vi "Dashboard Main.vi"() -> ()   [LabVIEW 2013]
uses:
  <vilib>/event_ctls.llb/eventvkey.ctl
  <vilib>/Rock Robotics/WPI/Dashboard/WPI_DashboardLogging Global.vi
  <vilib>/Utility/config.llb/Write Key (String).vi
  <vilib>/Utility/config.llb/Write Key (I32).vi
  <vilib>/Utility/config.llb/Read Key (String).vi
  <vilib>/Utility/config.llb/NI_LVConfig.lvlib
panel:
  in  "Save to File":bool
  in  "Read from File":bool=TRUE
  out "Image Message":string="Timeout in Camera Communications"
  in  "Rec Mode":enum32{"Stop", "Record", "Playback"}(radio)
  in  "Dashboard Tab":T1(tab)=enum."Drivetrain"
  in  "Camera Settings":T2={"Frame Rate"=30, "Compression"=30, "Size"=1} {"Frame Rate" scale=1.0..30.0; "Size" items=["640x480", "320x240", "160x120"]}
  out "MotorSliders R":cluster{"MotorSlide1":dbl, "MotorSlide2":dbl} {"MotorSlide2" scale=-1.0..1.0 scale format="%#_2e"; "MotorSlide1" scale=-1.0..1.0 scale format="%#_2e"}
  out "MotorChart R":cluster{"Numeric":dbl, "Numeric":dbl}(graph)
  out "MotorSliders L":T3 {"MotorSlide4 2" scale=0.0..14.0 scale format="%#_2e"; "MotorSlide2" scale=-1.0..1.0 scale format="%#_2e"; "MotorSlide1" scale=-1.0..1.0 scale format="%#_2e"}
  out "MotorChart L":T4(graph)
  out "JS1 Z":dbl(slide) scale=-1.0..1.0 scale format="%#_2e"
  out "Joystick 1":cluster{"X":dbl, "Y":dbl}[](graph)
  out "JS Buttons 1":T5
  out "JS2 Z":dbl(slide) scale=-1.0..1.0 scale format="%#_2e"
  out "Joystick 2":cluster{"X":dbl, "Y":dbl}[](graph)
  out "JS Buttons 2":T5
  out "Mode":T6(ring)=enum.""
  out "Camera IP":string="0.0.0.11"
  in  "DB Camera Config":bool
  out "fps":dbl format="%#.1g"
  out "Mbps":dbl format="%#.1g"
  out "Mbps 2":bool
  out "LED 1":bool
  in  "String":string
  in  "Dial":i8(knob) scale=0.0..10.0
  in  "Slider 1":dbl(slide) scale=0.0..100.0
  in  "Checkbox 2":bool
  in  "Checkbox 1":bool
  in  "Test Slider":dbl(slide) scale=0.0..100.0 scale format="%#_3g"
  in  "On/Off":bool caption="Solenoid"
  in  "Test Name":u16(ring) items=["Select the test to run...", "Example Test", "-------------------------------", "List of tests is built in robot code.", "Replace with your own automated tests."]
  in  "Test Tree":string(tree)
  in  "Motor":cluster{"Value":dbl, "Enable":bool} {"Value" scale=-1.0..1.0 scale format="%#_3g"}
  out "Progress":T7 {"Test Progress" scale=0.0..100.0}
  in  "Rev/Fwd":cluster{"Forward":bool, "Reverse":bool}
  in  "Test Ring":u16(ring) items=["Auto", "Fixed indoor", "Fixed outdoor 1", "Fixed outdoor 2", "Fixed fluorescent 1", "Fixed fluorescent 2", "Hold current"]
  in  "Listbox":i32(listbox)
  out "Tree":string(tree)
  in  "MaxSuspend":dbl=200.0
  in  "MinMotorPower":dbl
  in  "MinJoystickChange":dbl=0.05
  in  "ShiftDelay":dbl=200.0
  in  "DeadZone":dbl=0.1
  out "Camera Image":T8(plugin-control)
  in  "Enable":bool
  # "Left"
  # "Front"
  # "Right"
  # "Battery"
  # "Customize by placing controls and indicators here and name to\nmatch Dashboard Variables on robot."
  # "This tab is a great place for autonomous settings and validation.\nCustomize by placing controls and indicators here and name to\nmatch Dashboard Variables on robot."
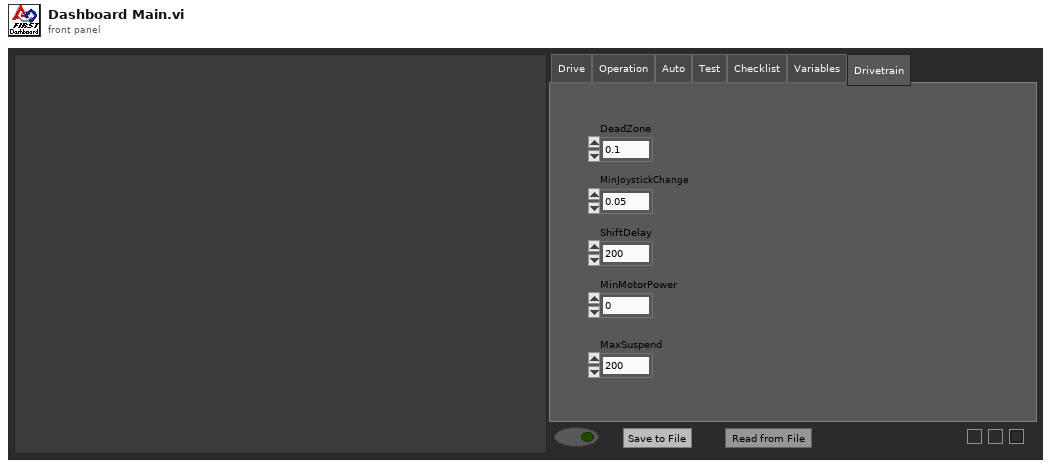
[diagram p1: front panel]
types:
  T1 = enum32{"Drive", "Operation", "Auto", "Test", "Checklist", "Variables", "Drivetrain"}
  T2 = cluster{"Frame Rate":i32, "Compression":i32, "Size":u16}
  T3 = cluster{"MotorSlide1":dbl, "MotorSlide2":dbl, "MotorSlide4 2":dbl}
  T4 = cluster{"Numeric":dbl, "Numeric":dbl, "Battery":sgl}
  T5 = cluster{bool, bool, bool, bool, bool, bool, bool, bool, bool, bool, bool, bool}
  T6 = enum8{"Tele-Op Disabled", "Tele-Op Enabled", "Auto Disabled", "Auto Enabled", "Test Disabled", "Test Enabled", ""}
  T7 = cluster{"Test Progress":u8, "Test Progress Text":string}
  T8 = typedef "IMAQ Image.ctl" = refnum<image>
  T9 = enum32{"Drive", "Operation", "Auto", "Test", "Checklist", "Variables", "DriveTrain"}
  T10 = enum32{"Drive", "Operation", "Auto", "Test", "Checklist", "Variables"}
  T11 = typedef "Image Type" = u32
  T12 = enum32{"Drive", "Operation", "Auto", "Test", "Checklist", "Variables", "DriveTrain"}[]
  T13 = typedef "NI_LVConfig.lvlib/Config Data RefNum.ctl" = refnum<k1>
  T14 = cluster{"Digital Inputs":bool[], "Digital Outputs":bool[]}
  T15 = cluster{"Competition mode":bool, "Robot Link":bool, "Autonomous":bool, "Enabled":bool, "E-Stop":bool, "Simulated":bool, "TestMode":bool, "Docked Window":bool}
  T16 = cluster{"Boolean Array[0]":bool, "Boolean Array[1]":bool, "Boolean Array[2]":bool, "Boolean Array[3]":bool, "Boolean Array[4]":bool, "Boolean Array[5]":bool, "Boolean Array[6]":bool, "Boolean Array[7]":bool, "Boolean Array[8]":bool, "Boolean Array[9]":bool, "Boolean Array[10]":bool, "Boolean Array[11]":bool}
  T17 = typedef "eventvkey.ctl" = enum16{"ASCII", "Enter", "Return", "Shift", "Ctrl", "Alt", "Cmd", "Opt", "Caps", "NumLock", "Clear", "Break", "Up", "Down", "Left", "Right", "Insert", "Delete", "Home", "End", "PageUp", "PageDown", "Escape", "Help", "Pause", "ScrollLock", "F1", "F2", "F3", "F4", "F5", "F6", "F7", "F8", "F9", "F10", "F11", "F12", "F13", "F14", "F15", "F16", "F17", "F18", "F19", "F20", "F21", "F22", "F23", "F24", "Play", "VolumeUp", "VolumeDown", "Mute", "Two Byte Char"}
  T18 = cluster{"Image Size":bool, "Image Type":bool, "Pixel Value":bool, "ROI Information":bool, "Zoom Factor":bool}
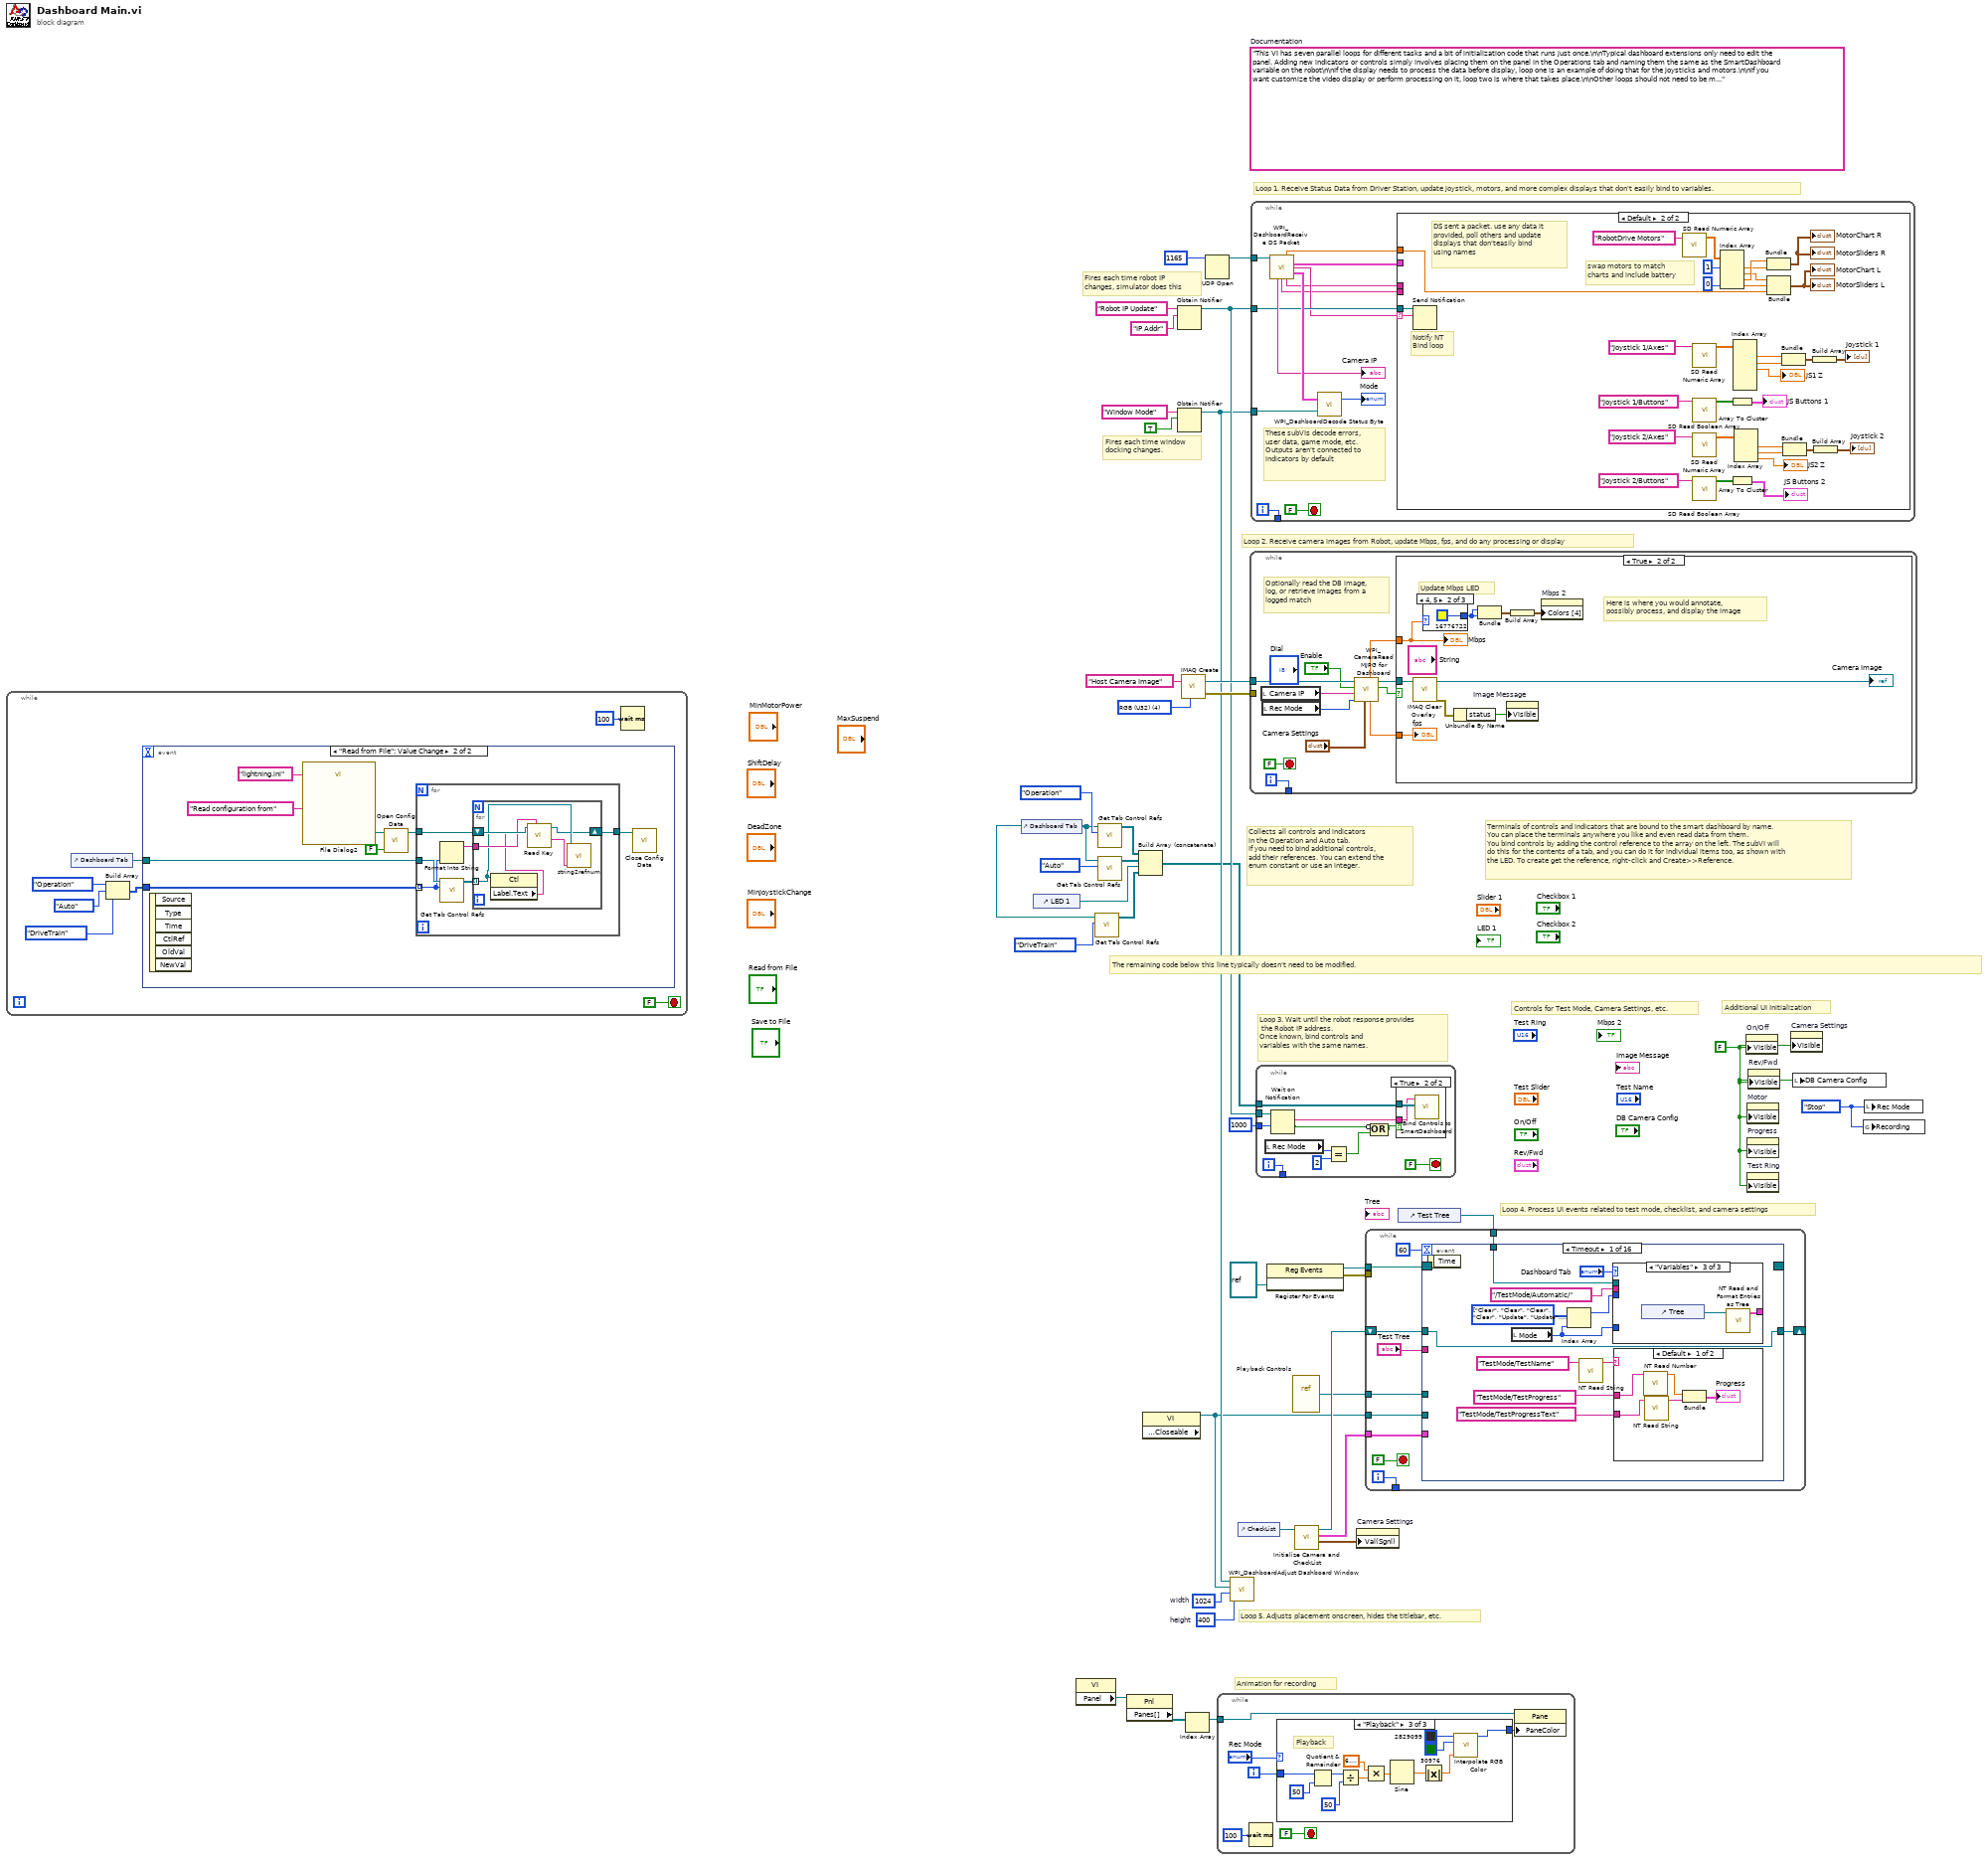
[diagram p0: block diagram]
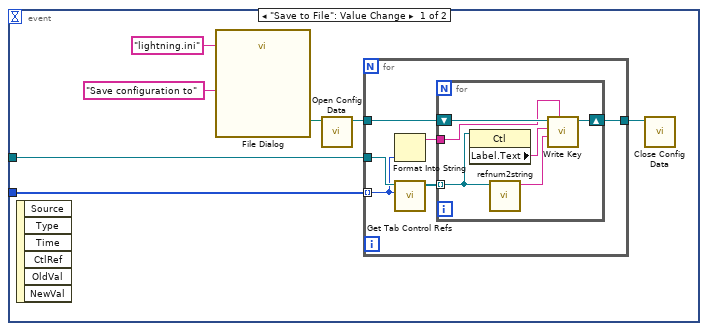
[diagram p2: hidden frame]
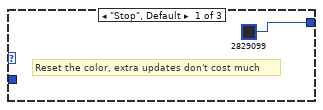
[diagram p3: hidden frame]
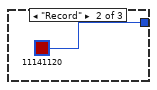
[diagram p4: hidden frame]
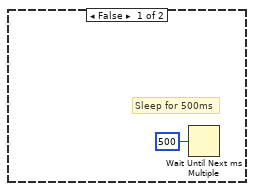
[diagram p6: hidden frame]
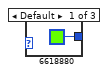
[diagram p7: hidden frame]
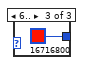
[diagram p8: hidden frame]
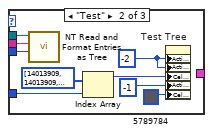
[diagram p10: hidden frame]
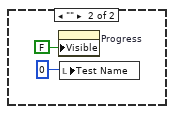
[diagram p11: hidden frame]
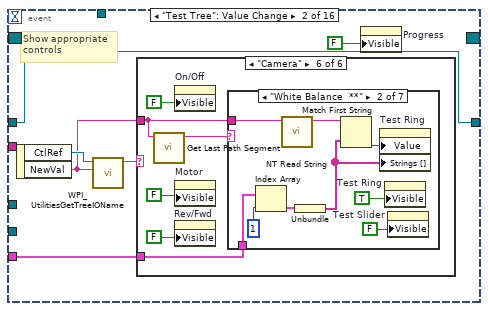
[diagram p12: hidden frame]
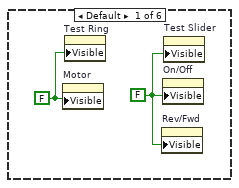
[diagram p13: hidden frame]
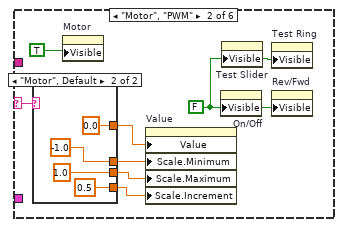
[diagram p14: hidden frame]
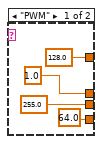
[diagram p15: hidden frame]
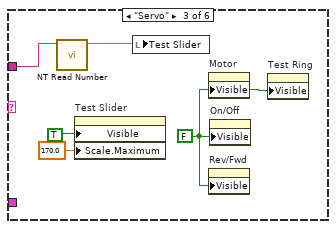
[diagram p16: hidden frame]
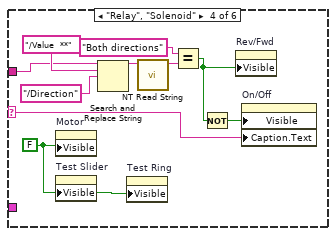
[diagram p17: hidden frame]
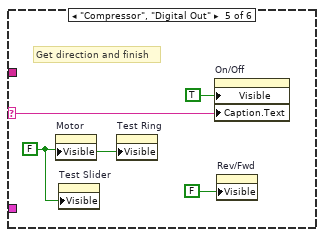
[diagram p18: hidden frame]
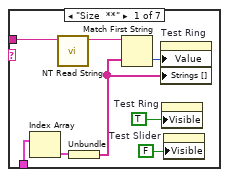
[diagram p19: hidden frame]
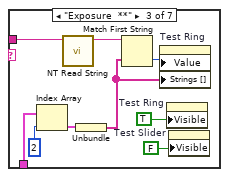
[diagram p20: hidden frame]
diagram:
  w10 = enum32{"Stop", "Record", "Playback"}."Stop" ("Rec Mode")
  w13 = 400  # height
  w14 = 1024  # width
  w27 = FALSE ("Visible")
  (unwired) "This VI has seven parallel loops for different tasks and a bit of initialization code that runs just once.\n\nTypical dashboard extensions only need to edit the panel. Adding new indicators or controls simply involves placing them on the panel in the Operations tab and naming them the same as the SmartDashboard variable on the robot\n\nIf the display needs to process the data before display, loop one is an example of doing that for the joysticks and motors.\n\nIf you want customize the video display or perform processing on it, loop two is where that takes place.\n\nOther loops should not need to be modified. They are pretty standard, and document the task they perform."  # Documentation
  w37 = T11 4 items=["Grayscale (U8)", "Grayscale (I16)", "Grayscale (SGL)", "Complex (CSG)", "RGB (U32)", "HSL (U32)", "RGB (U64)"] ("Image Type")
  # "Controls for Test Mode, Camera Settings, etc."
  # "Additional UI Initialization"
  # "Animation for recording"
  # "Fires each time robot IP\nchanges, simulator does this"
  # "Fires each time window\ndocking changes."
  # "Collects all controls and indicators\nin the Operation and Auto tab.\nIf you need to bind additional controls,\nadd their references. You can extend the\nenum constant or use an integer."
  # "The remaining code below this line typically doesn't need to be modified."
  # "Loop 4. Process UI events related to test mode, checklist, and camera settings"
  # "Terminals of controls and indicators that are bound to the smart dashboard by name.\nYou can place the terminals anywhere you like and even read data from them.\nYou bind controls by adding the control reference to the array on the left. The subVI will\ndo this for the contents of a tab, and you can do it for individual items too, as shown with\nthe LED. To create get the reference, right-click and Create>>Reference."
  # "Loop 3. Wait until the robot response provides\n the Robot IP address.\nOnce known, bind controls and\nvariables with the same names."
  # "Loop 5. Adjusts placement onscreen, hides the titlebar, etc."
  # "Loop 1. Receive Status Data from Driver Station, update joystick, motors, and more complex displays that don't easily bind to variables."
  # "Loop 2. Receive camera images from Robot, update Mbps, fps, and do any processing or display"
  n1 = while {
    stop <- FALSE stop-if-true
    n2 = control-ref of="Dashboard Tab"() -> (w43:refnum<vi>)
    n3 = Build Array(T10."Operation" ("Dashboard Tab"), T10."Auto" ("Dashboard Tab"), T9."DriveTrain" ("element")) -> (w44:T12)
    n4 = event shown="[1] \"Read from File\": Value Change" {
      selector: _ -> [_ _]
      dyn-events: _ -> [_ _]
      timeout: _ -> [_ _]
      tunnel: w44 -> [w53 w73]
      tunnel: w43 -> [w52 w72]
      event "Save to File": Value Change {
        n5 = event-data() -> ()  [unwired: 1 in, 6 out]
        n6 = call "File Dialog"("prompt"="Save configuration to", "default name"="lightning.ini") -> ("selected path"=w49:path)  [unwired: 10 in, 3 out]
        n7 = call <vilib>:"Open Config Data.vi"("configuration file path"=w49) -> ("refnum"=w51:T13)  [unwired: 8 in, 2 out]
        n8 = for {
          tunnel: w53 -> [w56] mode=indexing
          tunnel: w52 -> [w59]
          tunnel: w51 -> [w57]
          tunnel: [w54] -> w50
          n9 = Format Into String(w56) -> (resulting string=w55:string)  [unwired: 3 in, 1 out]
          n10 = call <vilib>:"Get Tab Control Refs.vi"("Page Index"=w56, "TabControl in"=w59) -> ("ControlsOnPage"=w58:refnum<vi>[])  [unwired: 9 in]
          n11 = for {
            tunnel: w58 -> [w64] mode=indexing
            tunnel: w55 -> [w62]
            shift-right: [w60] -> w54
            shift-left: w57 -> [w65]
            n12 = property class="Ctl"(reference=w64) -> ("Label.Text"=w63:string)  [unwired: 1 in, 2 out]
            n13 = call "refnum2string.vi"("Control in"=w64) -> ("String"=w61:string)  [unwired: 10 in]
            n14 = call-poly <vilib>:"Write Key.vi"("section"=w62, "value"=w61, "key"=w63, "refnum"=w65) -> ("refnum out"=w60:T13)  [unwired: 5 in, 2 out]
          }
        }
        n15 = call <vilib>:"Close Config Data.vi"("refnum"=w50) -> ()  [unwired: 9 in, 2 out]
      }
      event "Read from File": Value Change {
        n16 = event-data() -> ()  [unwired: 1 in, 6 out]
        n17 = call "File Dialog2"("prompt"="Read configuration from", "default name"="lightning.ini") -> ("selected path"=w69:path)  [unwired: 10 in, 3 out]
        n18 = call <vilib>:"Open Config Data.vi"("create file if necessary (T)"=FALSE, "configuration file path"=w69) -> ("refnum"=w71:T13)  [unwired: 7 in, 2 out]
        n19 = for {
          tunnel: w73 -> [w76] mode=indexing
          tunnel: w72 -> [w79]
          tunnel: w71 -> [w77]
          tunnel: [w74] -> w70
          n20 = Format Into String(w76) -> (resulting string=w75:string)  [unwired: 3 in, 1 out]
          n21 = call <vilib>:"Get Tab Control Refs.vi"("Page Index"=w76, "TabControl in"=w79) -> ("ControlsOnPage"=w78:refnum<vi>[])  [unwired: 9 in]
          n22 = for {
            tunnel: w78 -> [w81] mode=indexing
            tunnel: w75 -> [w84]
            shift-right: [w80] -> w74
            shift-left: w77 -> [w85]
            n23 = property class="Ctl"(reference=w81) -> ("Label.Text"=w83:string)  [unwired: 1 in, 2 out]
            n24 = call-poly <vilib>:"Read Key.vi"("section"=w84, "key"=w83, "refnum"=w85) -> ("value"=w82:string, "refnum out"=w80:T13)  [unwired: 5 in, 2 out]
            n25 = call "string2refnum.vi"("String"=w82, "Control in"=w81) -> ()  [unwired: 9 in]
          }
        }
        n26 = call <vilib>:"Close Config Data.vi"("refnum"=w70) -> ()  [unwired: 9 in, 2 out]
      }
    }
    n27 = Wait (ms)(milliseconds to wait=u32 100) -> ()  [unwired: 1 out]
  }
  n28 = control-ref of="Dashboard Tab"() -> (w2:refnum<vi>)
  n29 = control-ref of="LED 1"() -> (w5:refnum<vi>)
  n30 = property class="VI"() -> ("Panel"=w21:refnum<vi>)  [unwired: 2 in, 2 out]
  n31 = call <vilib>:"Get Tab Control Refs.vi"("Page Index"=T9."DriveTrain" ("element"), "TabControl in"=w2) -> ("ControlsOnPage"=w1:refnum<vi>[])  [unwired: 9 in]
  n32 = call <vilib>:"Get Tab Control Refs.vi"("Page Index"=T10."Operation" ("Dashboard Tab"), "TabControl in"=w2) -> ("ControlsOnPage"=w7:refnum<vi>[])  [unwired: 9 in]
  n33 = call <vilib>:"Get Tab Control Refs.vi"("Page Index"=T10."Auto" ("Dashboard Tab"), "TabControl in"=w2) -> ("ControlsOnPage"=w8:refnum<vi>[])  [unwired: 9 in]
  n34 = property class="Pnl"(reference=w21) -> ("Panes[]"=w22:refnum<vi>[])  [unwired: 1 in, 2 out]
  n35 = Build Array (concatenate)(w7, w8, w5, w1) -> (w4:refnum<vi>[])
  n36 = property class="VI" props=["Front Panel.Closeable"]() -> (reference out=w9:refnum<vi>)  [unwired: 2 in, 2 out]
  n37 = Obtain Notifier(name (unnamed)="Robot IP Update", notification data type="IP Addr" ("name (unnamed)")) -> (notifier out=w31:refnum<notifier>)  [unwired: 2 in, 2 out]
  n38 = Obtain Notifier(name (unnamed)="Window Mode", notification data type=TRUE) -> (notifier out=w12:refnum<notifier>)  [unwired: 2 in, 2 out]
  n39 = call "IMAQ Create"("Image Name"="Host Camera Image", "Image Type"=w37) -> ("New Image"=w35:T8, "error out"=w34:errorcluster)  [unwired: 2 in, 1 out]
  n40 = Index Array(array=w22) -> (element=w20:refnum<vi>)  [unwired: 1 in]
  n41 = UDP Open(11:u16 1165 ("port")) -> (port=w38:refnum<k16>)  [unwired: 2 in, 4 out]
  n42 = while {
    tunnel: w20 -> [w87]
    i -> [w90]
    stop <- FALSE stop-if-true
    n43 = Wait (ms)(milliseconds to wait=u32 100) -> ()  [unwired: 1 out]
    n44 = case shown="\"Playback\"" "Rec Mode" {
      tunnel: w90 -> [_ _ w105]
      tunnel: [u32 2829099 ("Base Color") u32 11141120 ("Target Color") w94] -> w86
      frame "Stop", Default {
        # "Reset the color, extra updates don't cost much"
      }
      frame "Record" {
      }
      frame "Playback" {
        # "Playback"
        n45 = Quotient & Remainder(x=w105, y=u32 50 ("milliseconds to wait")) -> (x-y*floor(x/y)=w101:u32)  [unwired: 1 out]
        n46 = Divide(x=w101, y=u32 50 ("milliseconds to wait")) -> (x/y=w98:dbl)
        n47 = Multiply(x=6.283185307179586, y=w98) -> (x*y=w103:dbl)
        n48 = Sine(x=w103) -> (sin(x)=w102:dbl)
        n49 = Absolute Value(x=w102) -> (abs(x)=w95:dbl)
        n50 = call "Interpolate RGB Color.vi"("Proportion"=w95, "Target Color"=u32 30976, "Base Color"=u32 2829099) -> ("Result Color"=w94:u32)  [unwired: 8 in]
      }
    }
    n51 = property class="Pane"(reference=w87, "PaneColor"=w86) -> ()  [unwired: 1 in, 2 out]
  }
  n52 = call <vilib>:"WPI_DashboardAdjust Dashboard Window.vi"("height"=w13, "width"=w14, "reference in"=w9, "Notifier in"=w12) -> ()  [unwired: 8 in]
  n53 = control-ref of="CheckList"() -> (w11:refnum<vi>)
  n54 = while {
    tunnel: w35 -> [w114]
    tunnel: w34 -> [_]
    tunnel: [w115] -> _
    i -> [w115]
    stop <- FALSE stop-if-true
    # "Optionally read the DB image,\nlog, or retrieve images from a\nlogged match"
    n55 = local read "Camera IP"() -> (w107:string)
    n56 = local read "Rec Mode"() -> (w106:enum32{"Stop", "Record", "Playback"})
    n57 = call <vilib>:"WPI_CameraRead MJPG for Dashboard.vi"("Camera Settings"="Camera Settings", "Rec Mode"=w106, "Camera IP"=w107, "Enable"="Enable", "Refnum in"=w114) -> ("Active"=w111:bool, "Refnum out"=w113:T8, "FPS"=w110:dbl, "Bandwidth (Mbps)"=w109:dbl)  [unwired: 3 in]
    n58 = case shown="True" w111 {
      tunnel: w113 -> [_ w121]
      tunnel: w109 -> [_ w120]
      tunnel: w110 -> [_ w118]
      frame False {
        # "Sleep for 500ms"
        n59 = Wait Until Next ms Multiple(millisecond multiple=u32 500) -> ()  [unwired: 1 out]
      }
      frame True {
        # "Here is where you would annotate,\npossibly process, and display the image"
        # "Update Mbps LED"
        n60 = call "IMAQ Clear Overlay"("Image"=w121) -> ("error out"=w125:errorcluster, "Image Out"=→"Camera Image":T8)  [unwired: 2 in, 7 out]
        n61 = case shown="4, 5" w120 {
          tunnel: [u32 6618880 ("Color Box") u32 16776722 ("Color Box") u32 16716800 ("Color Box")] -> w122
          frame Default {
          }
          frame 4, 5 {
          }
          frame 6.. {
          }
        }
        n62 = Unbundle By Name(w125) -> ("status"=w126:bool)
        n63 = Bundle("Color Box"=w122, "Color Box"=w122) -> (w124:cluster{"Color Box":u32, "Color Box":u32})  [unwired: 1 out]
        n64 = property on="Image Message" class="Str"("Visible"=w126) -> ()  [unwired: 2 in, 2 out]
        n65 = Build Array(w124) -> (w123:cluster{"Color Box":u32, "Color Box":u32}[])
        n66 = property on="Mbps 2" class="Bool (strict)"("Colors [4]"=w123) -> ()  [unwired: 2 in, 2 out]
        "Mbps" <- w120
        "fps" <- w118
      }
    }
  }
  n67 = while {
    tunnel: w38 -> [w140]
    tunnel: w31 -> [w135]
    tunnel: w12 -> [w139]
    tunnel: [w136] -> _
    i -> [w136]
    stop <- FALSE stop-if-true
    # "These subVIs decode errors, user data, game mode, etc.\nOutputs aren't connected to indicators by default"
    n68 = call <vilib>:"WPI_DashboardReceive DS Packet.vi"("Recv Socket"=w140) -> ("Battery"=w130:sgl, "Driver Station"=w131:T14, "Robot IP Address"=w134:string, "Status"=w141:T15, "Camera IP Address"=→"Camera IP":string, "Low Priority User Data"=w133:string, "High Priority User Data"=w132:string)  [unwired: 1 in, 7 out]
    n69 = call <vilib>:"WPI_DashboardDecode Status Byte.vi"("Window Mode Notifier"=w139, "Status"=w141) -> ("Mode"=→"Mode":T6)  [unwired: 1 out]
    n70 = case shown="Default" w134 {
      selector: w134 -> [_ w153]
      tunnel: w135 -> [_ w154]
      tunnel: w133 -> [_ _]
      tunnel: w132 -> [_ _]
      tunnel: w131 -> [_ _]
      tunnel: w130 -> [_ w152]
      frame "0.0.0.0" {
        # "DS not sending packets, or no robot exists yet.\nDon't poll the variables"
      }
      frame Default {
        # "Notify NT\nBind loop"
        # "DS sent a packet. use any data it\nprovided, poll others and update\ndisplays that don'teasily bind\nusing names"
        # "swap motors to match\ncharts and include battery"
        n71 = Send Notification(notification=w153, notifier=w154) -> ()  [unwired: 1 in, 2 out]
        n72 = call <vilib>:"SD Read Numeric Array.vi"("Name"="RobotDrive Motors") -> ("Numeric Array"=w151:dbl[])  [unwired: 8 in, 2 out]
        n73 = call <vilib>:"SD Read Numeric Array.vi"("Name"="Joystick 1/Axes") -> ("Numeric Array"=w170:dbl[])  [unwired: 8 in, 2 out]
        n74 = call <vilib>:"SD Read Boolean Array.vi"("Name"="Joystick 1/Buttons") -> ("Boolean Array"=w172:bool[])  [unwired: 8 in, 2 out]
        n75 = call <vilib>:"SD Read Numeric Array.vi"("Name"="Joystick 2/Axes") -> ("Numeric Array"=w164:dbl[])  [unwired: 8 in, 2 out]
        n76 = call <vilib>:"SD Read Boolean Array.vi"("Name"="Joystick 2/Buttons") -> ("Boolean Array"=w163:bool[])  [unwired: 8 in, 2 out]
        n77 = Index Array(array=w151, index #1=1, index #4=0) -> (element #1=w147:dbl, element #2=w146:dbl, element #3=w148:dbl, element #4=w143:dbl)  [unwired: 2 in]
        n78 = Array To Cluster(array=w172) -> (cluster=→"JS Buttons 1":T16)
        n79 = Array To Cluster(array=w163) -> (cluster=→"JS Buttons 2":T16)
        n80 = Index Array(array=w170) -> (element #1=w167:dbl, element #2=w168:dbl, element #3=→"JS1 Z":dbl)  [unwired: 6 in, 3 out]
        n81 = Index Array(array=w164) -> (element #1=w159:dbl, element #2=w158:dbl, element #3=→"JS2 Z":dbl)  [unwired: 3 in]
        n82 = Bundle("Numeric"=w148, "Numeric"=w147) -> (→"MotorChart R" →"MotorSliders R":cluster{"Numeric":dbl, "Numeric":dbl})  [unwired: 1 in]
        n83 = Bundle("Numeric"=w146, "Numeric"=w143, "Battery"=w152) -> (→"MotorChart L" →"MotorSliders L":T4)  [unwired: 1 in]
        n84 = Bundle("Numeric"=w167, "Numeric"=w168) -> (w166:cluster{"Numeric":dbl, "Numeric":dbl})  [unwired: 1 in]
        n85 = Bundle("Numeric"=w159, "Numeric"=w158) -> (w160:cluster{"Numeric":dbl, "Numeric":dbl})  [unwired: 1 in]
        n86 = Build Array(w166) -> (→"Joystick 1":cluster{"Numeric":dbl, "Numeric":dbl}[])
        n87 = Build Array(w160) -> (→"Joystick 2":cluster{"Numeric":dbl, "Numeric":dbl}[])
      }
    }
  }
  n88 = while {
    tunnel: w4 -> [w186]
    tunnel: w31 -> [w184]
    tunnel: [w182] -> _
    tunnel: u32 1000 ("milliseconds to wait") -> [w181]
    i -> [w182]
    stop <- FALSE stop-if-true
    n89 = local read "Rec Mode"() -> (w177:enum32{"Stop", "Record", "Playback"})
    n90 = Wait on Notification(notifier=w184, timeout in ms (-1)=w181) -> (notification=w183:string, timed out?=w179:bool)  [unwired: 2 in, 2 out]
    n91 = Equal?(x=w177, y=u16 2 ("Rec Mode")) -> (x = y?=w178:bool)
    n92 = Compound Arithmetic op=OR(invert w179, w178) -> (w180:bool)
    n93 = case shown="True" w180 {
      tunnel: w186 -> [_ w188]
      tunnel: w183 -> [_ w187]
      frame False {
      }
      frame True {
        n94 = call <vilib>:"Bind Controls to SmartDashboard.vi"("Bound Control Refs"=w188, "Server IP Address"=w187) -> ()  [unwired: 10 in]
      }
    }
  }
  n95 = register-events(refnum<vi> refnum) -> (reference out=w18:refnum<event-registration>, error out=w17:errorcluster)  [unwired: 2 in]
  n96 = vi-ref "Playback Controls.vi"() -> (w19:refnum<vi>)
  n97 = call "Initialize Camera and CheckList.vi"("ListBox in"=w11) -> ("Cluster"=w25:cluster{"value":i32, "value":i32, "index":i32}, "Array"=w26:cluster{string[]}[], "File Refnum"=w24:T13)  [unwired: 8 in]
  n98 = property on="Camera Settings" class="Clust (strict)"("Val(Sgnl)"=w25) -> ()  [unwired: 2 in, 2 out]
  n99 = control-ref of="Test Tree"() -> (w23:refnum<vi>)
  n100 = while {
    tunnel: w26 -> [w196]
    shift-right: [w195] -> _
    shift-left: w24 -> [w194]
    tunnel: [w193] -> _
    tunnel: w23 -> [w192]
    tunnel: w19 -> [w191]
    tunnel: w18 -> [w190]
    tunnel: w17 -> [_]
    tunnel: w9 -> [w189]
    i -> [w193]
    stop <- FALSE stop-if-true
    n101 = event shown="[0] Timeout" {
      selector: w190 -> [_ _ _ _ _ _ _ _ _ _ _ _ _ _ _ _]
      dyn-events: [_ _ _ _ _ _ _ _ _ _ _ _ _ w434 _ _] -> _
      timeout: u32 60 ("milliseconds to wait") -> [_ _ _ _ _ _ _ _ _ _ _ _ _ _ _ _]
      tunnel: w192 -> [w206 _ _ _ _ _ _ _ _ _ _ _ _ _ _ _]
      tunnel: "Test Tree" -> [_ _ _ _ _ _ _ _ w403 w411 w413 w417 w425 _ _ _]
      tunnel: w196 -> [_ w230 _ _ _ _ w367 w397 _ _ _ _ _ _ _ _]
      tunnel: [w200 w229 w328 w333 w341 w353 w366 w390 w402 w409 w412 w416 w424 w436 w450 w451] -> w195
      tunnel: w194 -> [w200 w229 w328 w333 w341 w353 w365 w390 w402 w409 w412 w416 w424 w436 w450 w451]
      tunnel: w191 -> [_ _ _ _ _ _ _ _ _ _ _ _ _ w437 _ w454]
      tunnel: w189 -> [_ _ _ _ _ _ _ _ _ _ _ _ _ w432 _ _]
      event Timeout {
        w205 = enum16{"Update", "Clear"}[] [enum."Clear", enum."Clear", enum."Clear", enum."Clear", enum."Update", enum."Update", enum."Clear"] items=["Update", "Clear"]
        n102 = event-data() -> ()  [unwired: 1 in, 1 out]
        n103 = local read "Mode"() -> (w203:T6)
        n104 = Index Array(array=w205, index=w203) -> (element=w204:enum16{"Update", "Clear"})
        n105 = call <vilib>:"NT Read String.vi"("Name"="TestMode/TestName") -> ("String"=w209:string)  [unwired: 9 in, 1 out]
        n106 = case shown="\"Variables\"" "Dashboard Tab" {
          tunnel: w206 -> [_ w219 _]
          tunnel: "/TestMode/Automatic/" ("Name Pattern") -> [_ w218 _]
          tunnel: w204 -> [_ w217 _]
          tunnel: w203 -> [_ w215 _]
          tunnel: [_ _ w221] -> _
          frame "Operation", Default {
          }
          frame "Test" {
            w214 = -2 ("Active Item:Row Number")
            n107 = call <vilib>:"NT Read and Format Entries as Tree.vi"("Operation"=w217, "Name Pattern"=w218, "Tree Refnum"=w219) -> ()  [unwired: 7 in, 2 out]
            n108 = Index Array(array=u32[] [14013909, 14013909, 14013909, 14013909, 14013909, 16777215, 14013909], index=w215) -> (element=w213:u32)
            n109 = property on="Test Tree" class="Tree (strict)"("Active Item Row Number"=w214, "ActiveColNum"=w214, "CellBG"=w213, "Active Item Row Number"=-1 ("Active Item:Row Number"), "CellBG"=u32 5789784 ("Color Box")) -> ()  [unwired: 2 in, 2 out]
          }
          frame "Variables" {
            n110 = control-ref of="Tree"() -> (w220:refnum<vi>)
            n111 = call <vilib>:"NT Read and Format Entries as Tree.vi"("Tree Refnum"=w220) -> ("Formatted Strings"=w221:cluster{"Name":string, "Value":string}[])  [unwired: 9 in, 1 out]
          }
        }
        n112 = case shown="Default" w209 {
          tunnel: "TestMode/TestProgress" ("Name") -> [w223 _]
          tunnel: "TestMode/TestProgressText" ("Name") -> [w222 _]
          frame Default {
            n113 = call <vilib>:"NT Read Number.vi"("Name"=w223) -> ("Numeric"=w224:dbl)  [unwired: 9 in, 1 out]
            n114 = call <vilib>:"NT Read String.vi"("Name"=w222) -> ("String"=w225:string)  [unwired: 9 in, 1 out]
            n115 = Bundle("Numeric"=w224, "String"=w225) -> (→"Progress":cluster{"Numeric":dbl, "String":string})  [unwired: 1 in]
          }
          frame "" {
            n116 = property on="Progress" class="Clust (strict)"("Visible"=FALSE) -> ()  [unwired: 2 in, 2 out]
            n117 = local write "Test Name"(u16 0) -> ()
          }
        }
      }
      event "Test Tree": Value Change {
        # "Show appropriate\ncontrols"
        n118 = event-data() -> ("CtlRef"=w233:refnum<vi>, "NewVal"=w231:string)  [unwired: 1 in]
        n119 = call <vilib>:"WPI_UtilitiesGetTreeIOName.vi"("NewVal"=w231, "TreeControl in"=w233) -> ("I/O Name"=w234:string)  [unwired: 9 in]
        n120 = case shown="\"Camera\"" w234 {
          selector: w234 -> [_ w241 _ w259 w268 _]
          tunnel: w231 -> [_ _ w256 w258 _ w275]
          tunnel: w230 -> [_ _ _ _ _ w274]
          frame Default {
            w236 = FALSE ("Visible")
            w235 = FALSE ("Visible")
            n121 = property on="Motor" class="Clust (strict)"("Visible"=w235) -> ()  [unwired: 2 in, 2 out]
            n122 = property on="Test Ring" class="Ring (strict)"("Visible"=w235) -> ()  [unwired: 2 in, 2 out]
            n123 = property on="Rev/Fwd" class="Clust (strict)"("Visible"=w236) -> ()  [unwired: 2 in, 2 out]
            n124 = property on="On/Off" class="Bool (strict)"("Visible"=w236) -> ()  [unwired: 2 in, 2 out]
            n125 = property on="Test Slider" class="Slide (strict)"("Visible"=w236) -> ()  [unwired: 2 in, 2 out]
          }
          frame "Motor", "PWM" {
            w242 = FALSE ("Visible")
            n126 = case shown="\"Motor\", Default" w241 {
              tunnel: [1.0 ("Value") -1.0 ("Value")] -> w240
              tunnel: [255.0 ("Value") 1.0 ("Value")] -> w239
              tunnel: [128.0 ("Value") 0.0 ("Value")] -> w238
              tunnel: [64.0 ("Value") 0.5 ("Value")] -> w237
              frame "PWM" {
              }
              frame "Motor", Default {
              }
            }
            n127 = property on="Motor" class="Clust (strict)"("Visible"=TRUE) -> ()  [unwired: 2 in, 2 out]
            n128 = property on="Value" class="Slide (strict)"("Value"=w238, "Scale.Minimum"=w240, "Scale.Maximum"=w239, "Scale.Increment"=w237) -> ()  [unwired: 2 in, 2 out]
            n129 = property on="On/Off" class="Bool (strict)"("Visible"=w242) -> ()  [unwired: 2 in, 2 out]
            n130 = property on="Test Slider" class="Slide (strict)"("Visible"=w242) -> ()  [unwired: 2 in, 2 out]
            n131 = property on="Test Ring" class="Ring (strict)"("Visible"=w242) -> ()  [unwired: 2 in, 2 out]
            n132 = property on="Rev/Fwd" class="Clust (strict)"("Visible"=w242) -> ()  [unwired: 2 in, 2 out]
          }
          frame "Servo" {
            w254 = FALSE ("Visible")
            n133 = call <vilib>:"NT Read Number.vi"("Name"=w256) -> ("Numeric"=w255:dbl)  [unwired: 9 in, 1 out]
            n134 = property on="Test Slider" class="Slide (strict)"("Visible"=TRUE, "Scale.Maximum"=170.0 ("Scale.Range:Maximum")) -> ()  [unwired: 2 in, 2 out]
            n135 = local write "Test Slider"(w255) -> ()
            n136 = property on="Motor" class="Clust (strict)"("Visible"=w254) -> ()  [unwired: 2 in, 2 out]
            n137 = property on="Rev/Fwd" class="Clust (strict)"("Visible"=w254) -> ()  [unwired: 2 in, 2 out]
            n138 = property on="On/Off" class="Bool (strict)"("Visible"=w254) -> ()  [unwired: 2 in, 2 out]
            n139 = property on="Test Ring" class="Ring (strict)"("Visible"=w254) -> ()  [unwired: 2 in, 2 out]
          }
          frame "Relay", "Solenoid" {
            w257 = FALSE ("Visible")
            n140 = property on="Motor" class="Clust (strict)"("Visible"=w257) -> ()  [unwired: 2 in, 2 out]
            n141 = property on="Test Slider" class="Slide (strict)"("Visible"=w257) -> ()  [unwired: 2 in, 2 out]
            n142 = Search and Replace String(input string=w258, search string="/Value  **", replace string="/Direction") -> (result string=w264:string)  [unwired: 5 in, 3 out]
            n143 = property on="Test Ring" class="Ring (strict)"("Visible"=w257) -> ()  [unwired: 2 in, 2 out]
            n144 = call <vilib>:"NT Read String.vi"("Name"=w264) -> ("String"=w262:string)  [unwired: 9 in, 1 out]
            n145 = Equal?(x="Both directions", y=w262) -> (x = y?=w260:bool)
            n146 = Not(x=w260) -> (.not. x?=w261:bool)
            n147 = property on="Rev/Fwd" class="Clust (strict)"("Visible"=w260) -> ()  [unwired: 2 in, 2 out]
            n148 = property on="On/Off" class="Bool (strict)"("Visible"=w261, "Caption.Text"=w259) -> ()  [unwired: 2 in, 2 out]
          }
          frame "Compressor", "Digital Out" {
            w267 = FALSE ("Visible")
            # "Get direction and finish"
            n149 = property on="Motor" class="Clust (strict)"("Visible"=w267) -> ()  [unwired: 2 in, 2 out]
            n150 = property on="Test Slider" class="Slide (strict)"("Visible"=w267) -> ()  [unwired: 2 in, 2 out]
            n151 = property on="Test Ring" class="Ring (strict)"("Visible"=w267) -> ()  [unwired: 2 in, 2 out]
            n152 = property on="On/Off" class="Bool (strict)"("Visible"=TRUE, "Caption.Text"=w268) -> ()  [unwired: 2 in, 2 out]
            n153 = property on="Rev/Fwd" class="Clust (strict)"("Visible"=FALSE) -> ()  [unwired: 2 in, 2 out]
          }
          frame "Camera" {
            n154 = call <vilib>:"Get Last Path Segment.vi"("String in"=w275) -> ("String out"=w276:string)  [unwired: 10 in]
            n155 = property on="On/Off" class="Bool (strict)"("Visible"=FALSE) -> ()  [unwired: 2 in, 2 out]
            n156 = property on="Motor" class="Clust (strict)"("Visible"=FALSE) -> ()  [unwired: 2 in, 2 out]
            n157 = property on="Rev/Fwd" class="Clust (strict)"("Visible"=FALSE) -> ()  [unwired: 2 in, 2 out]
            n158 = case shown="\"White Balance  **\"" w276 {
              tunnel: w275 -> [w282 w291 w300 w309 w318 _ w324]
              tunnel: w274 -> [w280 w288 w297 w306 w315 _ _]
              frame "Size  **" {
                n159 = Index Array(array=w280) -> (element=w279:cluster{string[]})  [unwired: 1 in]
                n160 = call <vilib>:"NT Read String.vi"("Name"=w282) -> ("String"=w281:string)  [unwired: 9 in, 1 out]
                n161 = Unbundle(w279) -> (w277:string[])
                n162 = Match First String(2:w277, 3:w281) -> (0:w278:i32)  [unwired: 1 out]
                n163 = property on="Test Ring" class="Ring (strict)"("Value"=w278, "Strings []"=w277) -> ()  [unwired: 2 in, 2 out]
                n164 = property on="Test Ring" class="Ring (strict)"("Visible"=TRUE) -> ()  [unwired: 2 in, 2 out]
                n165 = property on="Test Slider" class="Slide (strict)"("Visible"=FALSE) -> ()  [unwired: 2 in, 2 out]
              }
              frame "White Balance  **" {
                n166 = Index Array(array=w288, index=1) -> (element=w289:cluster{string[]})
                n167 = call <vilib>:"NT Read String.vi"("Name"=w291) -> ("String"=w290:string)  [unwired: 9 in, 1 out]
                n168 = Unbundle(w289) -> (w286:string[])
                n169 = Match First String(2:w286, 3:w290) -> (0:w285:i32)  [unwired: 1 out]
                n170 = property on="Test Ring" class="Ring (strict)"("Value"=w285, "Strings []"=w286) -> ()  [unwired: 2 in, 2 out]
                n171 = property on="Test Ring" class="Ring (strict)"("Visible"=TRUE) -> ()  [unwired: 2 in, 2 out]
                n172 = property on="Test Slider" class="Slide (strict)"("Visible"=FALSE) -> ()  [unwired: 2 in, 2 out]
              }
              frame "Exposure  **" {
                n173 = Index Array(array=w297, index=2) -> (element=w298:cluster{string[]})
                n174 = call <vilib>:"NT Read String.vi"("Name"=w300) -> ("String"=w299:string)  [unwired: 9 in, 1 out]
                n175 = Unbundle(w298) -> (w294:string[])
                n176 = Match First String(2:w294, 3:w299) -> (0:w295:i32)  [unwired: 1 out]
                n177 = property on="Test Ring" class="Ring (strict)"("Value"=w295, "Strings []"=w294) -> ()  [unwired: 2 in, 2 out]
                n178 = property on="Test Ring" class="Ring (strict)"("Visible"=TRUE) -> ()  [unwired: 2 in, 2 out]
                n179 = property on="Test Slider" class="Slide (strict)"("Visible"=FALSE) -> ()  [unwired: 2 in, 2 out]
              }
              frame "Exposure Priority  **" {
                n180 = Index Array(array=w306, index=3) -> (element=w307:cluster{string[]})
                n181 = call <vilib>:"NT Read String.vi"("Name"=w309) -> ("String"=w308:string)  [unwired: 9 in, 1 out]
                n182 = Unbundle(w307) -> (w303:string[])
                n183 = Match First String(2:w303, 3:w308) -> (0:w304:i32)  [unwired: 1 out]
                n184 = property on="Test Ring" class="Ring (strict)"("Value"=w304, "Strings []"=w303) -> ()  [unwired: 2 in, 2 out]
                n185 = property on="Test Ring" class="Ring (strict)"("Visible"=TRUE) -> ()  [unwired: 2 in, 2 out]
                n186 = property on="Test Slider" class="Slide (strict)"("Visible"=FALSE) -> ()  [unwired: 2 in, 2 out]
              }
              frame "Color Enable  **" {
                n187 = Index Array(array=w315, index=4) -> (element=w316:cluster{string[]})
                n188 = call <vilib>:"NT Read String.vi"("Name"=w318) -> ("String"=w317:string)  [unwired: 9 in, 1 out]
                n189 = Unbundle(w316) -> (w312:string[])
                n190 = Match First String(2:w312, 3:w317) -> (0:w313:i32)  [unwired: 1 out]
                n191 = property on="Test Ring" class="Ring (strict)"("Value"=w313, "Strings []"=w312) -> ()  [unwired: 2 in, 2 out]
                n192 = property on="Test Ring" class="Ring (strict)"("Visible"=TRUE) -> ()  [unwired: 2 in, 2 out]
                n193 = property on="Test Slider" class="Slide (strict)"("Visible"=FALSE) -> ()  [unwired: 2 in, 2 out]
              }
              frame Default {
                n194 = property on="Test Ring" class="Ring (strict)"("Visible"=FALSE) -> ()  [unwired: 2 in, 2 out]
                n195 = property on="Test Slider" class="Slide (strict)"("Visible"=FALSE) -> ()  [unwired: 2 in, 2 out]
              }
              frame "Brightness  **", "Color Level  **", "Compression  **", "FPS  **", "Sharpness  **" {
                n196 = call <vilib>:"NT Read Number.vi"("Name"=w324) -> ("Numeric"=w323:dbl)  [unwired: 9 in, 1 out]
                n197 = local write "Test Slider"(w323) -> ()
                n198 = property on="Test Slider" class="Slide (strict)"("Visible"=TRUE, "Scale.Maximum"=100.0 ("Scale.Range:Maximum")) -> ()  [unwired: 2 in, 2 out]
                n199 = property on="Test Ring" class="Ring (strict)"("Visible"=FALSE) -> ()  [unwired: 2 in, 2 out]
              }
            }
          }
        }
        n200 = property on="Progress" class="Clust (strict)"("Visible"=FALSE) -> ()  [unwired: 2 in, 2 out]
      }
      event "Test Name": Mouse Enter {
        # "Populate the ring with the list of tests"
        n201 = event-data() -> ()  [unwired: 1 in, 1 out]
        n202 = call <vilib>:"NT Read String Array.vi"("Name"="TestMode/TestList") -> ("String Array"=w332:string[])  [unwired: 9 in, 1 out]
        n203 = Build Array (concatenate)("Select the test to run...", w332) -> (w331:string[])
        n204 = property on="Test Name" class="Ring (strict)"("Strings []"=w331) -> ()  [unwired: 2 in, 2 out]
      }
      event "Test Name": Value Change {
        w334 = FALSE ("Visible")
        # "Tell the robot the test name to run"
        n205 = event-data() -> ("NewVal"=w338:u16)  [unwired: 1 in]
        n206 = property on="Test Name" class="Ring (strict)"() -> ("Strings []"=w339:string[])  [unwired: 2 in, 2 out]
        n207 = local write "Progress"(T7 {"Test Progress"=0, "Test Progress Text"=""} ("Progress")) -> ()
        n208 = Index Array(array=w339, index=w338) -> (element=w337:string)
        n209 = call <vilib>:"NT Write String.vi"("String"=w337, "Name"="TestMode/TestName") -> ()  [unwired: 9 in, 1 out]
        n210 = property on="Progress" class="Clust (strict)"("Visible"=TRUE) -> ()  [unwired: 2 in, 2 out]
        n211 = property on="Motor" class="Clust (strict)"("Visible"=w334) -> ()  [unwired: 2 in, 2 out]
        n212 = property on="Test Slider" class="Slide (strict)"("Visible"=w334) -> ()  [unwired: 2 in, 2 out]
        n213 = property on="On/Off" class="Bool (strict)"("Visible"=w334) -> ()  [unwired: 2 in, 2 out]
        n214 = property on="Rev/Fwd" class="Clust (strict)"("Visible"=w334) -> ()  [unwired: 2 in, 2 out]
        n215 = property on="Test Ring" class="Ring (strict)"("Visible"=w334) -> ()  [unwired: 2 in, 2 out]
      }
      event "Listbox": Double Click {
        n216 = event-data() -> ("PlatMods.Shift"=w342:bool, "Row"=w344:i32)  [unwired: 1 in]
        n217 = case shown="True" w342 {
          tunnel: w344 -> [w348 _]
          tunnel: 1 -> [w347 _]
          frame False {
            n218 = property on="Listbox" class="LstBox (strict)"() -> ("Item Symbols"=w346:i32[])  [unwired: 2 in, 2 out]
            n219 = Replace Array Subset(array=w346, new element=w347, index=w348) -> (w345:i32[])
            n220 = property on="Listbox" class="LstBox (strict)"("Item Symbols"=w345) -> ()  [unwired: 2 in, 2 out]
          }
          frame True {
            w349 = 0 ("Top Row")
            n221 = property on="Listbox" class="LstBox (strict)"() -> ("Number of Rows"=w351:u32)  [unwired: 2 in, 2 out]
            n222 = Initialize Array(0, w351) -> (w350:i32[])
            n223 = property on="Listbox" class="LstBox (strict)"("Top Row"=w349, "Value"=w349, "Item Symbols"=w350) -> ()  [unwired: 2 in, 2 out]
          }
        }
      }
      event "Listbox": Key Down {
        n224 = event-data() -> ("VKey"=w355:T17)  [unwired: 1 in]
        n225 = case shown="\"Left\", \"Right\"" w355 {
          selector: w355 -> [w360 _]
          tunnel: eventvkey."Left" ("VKey") -> [w358 _]
          frame "Left", "Right" {
            n226 = Equal?(x=w358, y=w360) -> (x = y?=w359:bool)
            n227 = Select(t=0, s=w359, f=1) -> (s? t:f=w361:i32)
            n228 = property on="Listbox" class="LstBox (strict)"() -> ("Item Symbols"=w364:i32[])  [unwired: 2 in, 2 out]
            n229 = Replace Array Subset(array=w364, new element=w361, index="Listbox") -> (w363:i32[])
            n230 = property on="Listbox" class="LstBox (strict)"("Item Symbols"=w363) -> ()  [unwired: 2 in, 2 out]
          }
          frame Default {
          }
        }
      }
      event "DB Camera Config": Value Change {
        n231 = event-data() -> ("NewVal"=w368:bool)  [unwired: 1 in]
        n232 = case shown="False" w368 {
          tunnel: w367 -> [w377 _]
          tunnel: [w370 w388] -> w366
          tunnel: w365 -> [w369 w388]
          frame False {
            w384 = "Camera"
            w387 = FALSE ("Visible")
            n233 = local read "Camera Settings"() -> (w376:T2)
            n234 = Index Array(array=w377) -> (element=w380:cluster{string[]})  [unwired: 1 in]
            n235 = Unbundle(w376) -> ("Frame Rate"=w375:i32, "Compression"=w374:i32, "Size"=w378:u16)
            n236 = Unbundle(w380) -> (w379:string[])
            n237 = Index Array(array=w379, index=w378) -> (element=w373:string)
            n238 = call-poly <vilib>:"Write Key.vi"("section"=w384, "value"=w373, "key"="Size", "refnum"=w369) -> ("refnum out"=w386:T13)  [unwired: 2 in, 5 out]
            n239 = call-poly <vilib>:"Write Key.vi"("section"=w384, "value"=w375, "key"="FrameRate", "refnum"=w386) -> ("refnum out"=w385:T13)  [unwired: 1 in, 6 out]
            n240 = property on="Camera Settings" class="Clust (strict)"("Visible"=w387) -> ()  [unwired: 2 in, 2 out]
            n241 = local write "DB Camera Config"(w387) -> ()
            n242 = call-poly <vilib>:"Write Key.vi"("section"=w384, "value"=w374, "key"="Compression", "refnum"=w385) -> ("refnum out"=w371:T13)  [unwired: 1 in, 6 out]
            n243 = call <vilib>:"Close Config Data.vi"("refnum"=w371) -> ("file path"=w372:path)  [unwired: 2 in, 8 out]
            n244 = call <vilib>:"Open Config Data.vi"("configuration file path"=w372) -> ("refnum"=w370:T13)  [unwired: 8 in, 2 out]
          }
          frame True {
            n245 = property on="Camera Settings" class="Clust (strict)"("Visible"=TRUE) -> ()  [unwired: 2 in, 2 out]
          }
        }
      }
      event "Camera Settings": Value Change {
        n246 = event-data() -> ("NewVal"=w401:T2)  [unwired: 1 in]
        n247 = Index Array(array=w397) -> (element=w396:cluster{string[]})  [unwired: 1 in]
        n248 = Unbundle(w401) -> ("Frame Rate"=w392:i32, "Compression"=w391:i32, "Size"=w394:u16)
        n249 = Unbundle(w396) -> (w395:string[])
        n250 = Index Array(array=w395, index=w394) -> (element=w393:string)
        n251 = Format Into String(format string="%s   %dfps   %d%%", w393, w392, w391) -> (resulting string=w398:string)  [unwired: 2 in, 1 out]
        n252 = Build Array(w398) -> (w399:string[])
        n253 = property on="DB Camera Config" class="Bool (strict)"("Strings [4]"=w399) -> ()  [unwired: 2 in, 2 out]
      }
      event "Motor.Enable": Value Change {
        n254 = event-data() -> ("NewVal"=w407:bool)  [unwired: 1 in]
        n255 = Unbundle("Motor") -> ("Value"=w406:dbl)  [unwired: 1 out]
        n256 = Select(t=w406, s=w407, f=0.0) -> (s? t:f=w404:dbl)
        n257 = call <vilib>:"NT Write Number.vi"("Numeric"=w404, "Name"=w403) -> ()  [unwired: 9 in, 1 out]
      }
      event "Test Slider": Value Change {
        n258 = event-data() -> ("NewVal"=w410:dbl)  [unwired: 1 in]
        n259 = call <vilib>:"NT Write Number.vi"("Numeric"=w410, "Name"=w411) -> ()  [unwired: 9 in, 1 out]
      }
      event "On/Off": Value Change {
        n260 = event-data() -> ("NewVal"=w415:bool)  [unwired: 1 in]
        n261 = Boolean To (0,1)(Boolean=w415) -> (0, 1=w414:i16)
        n262 = call <vilib>:"NT Write Number.vi"("Numeric"=w414, "Name"=w413) -> ()  [unwired: 9 in, 1 out]
      }
      event "Rev/Fwd": Value Change {
        n263 = event-data() -> ("NewVal.Forward"=w423:bool, "NewVal.Reverse"=w422:bool)  [unwired: 1 in]
        n264 = Boolean To (0,1)(Boolean=w423) -> (0, 1=w419:i16)
        n265 = Boolean To (0,1)(Boolean=w422) -> (0, 1=w421:i16)
        n266 = Negate(x=w421) -> (-x=w420:i16)
        n267 = Add(x=w419, y=w420) -> (x+y=w418:i16)
        n268 = call <vilib>:"NT Write Number.vi"("Numeric"=w418, "Name"=w417) -> ()  [unwired: 9 in, 1 out]
      }
      event "Test Ring": Value Change {
        n269 = event-data() -> ("NewVal"=w427:u16)  [unwired: 1 in]
        n270 = property on="Test Ring" class="Ring (strict)"() -> ("Strings []"=w428:string[])  [unwired: 2 in, 2 out]
        n271 = Index Array(array=w428, index=w427) -> (element=w426:string)
        n272 = call <vilib>:"NT Write String.vi"("String"=w426, "Name"=w425) -> ()  [unwired: 9 in, 1 out]
      }
      event "Rec Mode": Value Change {
        # "Update globals for recording mode and path to read log from.\nClear when logging and let NetworkTables set path for vision to\nuse."
        n273 = event-data() -> ("NewVal"=w438:enum32{"Stop", "Record", "Playback"})  [unwired: 1 in]
        n274 = global write "WPI_DashboardLogging Global.vi" "Logging Filename"(path "") -> ()
        n275 = case shown="\"Stop\", \"Record\"" w438 {
          tunnel: w437 -> [_ w440 w448]
          tunnel: [_ _ w447] -> w434
          tunnel: [_ _ w446] -> _
          tunnel: w432 -> [_ _ w444]
          tunnel: cluster{i32, i32} {-250, 170} -> [_ _ w443]
          tunnel: [_ _ T18 {"Image Size"=TRUE, "Image Type"=TRUE, "Pixel Value"=TRUE, "ROI Information"=TRUE, "Zoom Factor"=FALSE} ("Image Information Shown:All Elements")] -> w430
          tunnel: [_ _ TRUE ("Zoom Factor")] -> w429
          frame Default {
          }
          frame "Stop", "Record" {
            # "Place Window too"
            n276 = invoke class="VI" method="FP.Close"(reference=w440) -> (reference out=w439:refnum<vi>)  [unwired: 2 in, 2 out]
            n277 = invoke class="VI" method="Abort VI"(reference=w439) -> ()  [unwired: 2 in, 3 out]
          }
          frame "Playback" {
            n278 = call "Open Playback Panel.vi"("Offset"=w443, "DB VI Ref"=w444, "Playback in"=w448) -> ("Playback out"=w445:refnum<vi>)  [unwired: 8 in]
            n279 = register-events(w445) -> (reference out=w447:refnum<event-registration>, error out=w446:errorcluster)  [unwired: 2 in]
          }
        }
        n280 = global write "WPI_DashboardLogging Global.vi" "Recording"(w438) -> ()
        n281 = property on="Camera Image" class="ImageControl"("Image Information Shown"=w430, "Image Information Visible"=w429) -> ()  [unwired: 2 in, 2 out]
        n282 = call <vilib>:"WPI_DashboardNT Log FieldName Cache.vi"("Operation"=enum16{"Lookup/Add", "Index", "Clear"}."Clear") -> ()  [unwired: 8 in, 3 out]
      }
      event Panel Close {
        w449 = enum32{"Stop", "Record", "Playback"}."Stop" ("Rec Mode")
        n283 = event-data() -> ()  [unwired: 1 in, 4 out]
        n284 = local write "Rec Mode"(w449) -> ()
        n285 = global write "WPI_DashboardLogging Global.vi" "Recording"(w449) -> ()
      }
      event Panel Close {
        # "Abort playback window and ourself"
        n286 = event-data() -> ()  [unwired: 1 in, 4 out]
        n287 = invoke class="VI" method="FP.Close"(reference=w454) -> (reference out=w453:refnum<vi>)  [unwired: 2 in, 2 out]
        n288 = invoke class="VI" method="Abort VI"(reference=w453) -> (error out=w452:errorcluster)  [unwired: 2 in, 2 out]
        n289 = invoke class="VI" method="Abort VI"(error in=w452) -> ()  [unwired: 2 in, 3 out]
      }
    }
  }
  n290 = property on="On/Off" class="Bool (strict)"("Visible"=w27) -> ()  [unwired: 2 in, 2 out]
  n291 = property on="Motor" class="Clust (strict)"("Visible"=w27) -> ()  [unwired: 2 in, 2 out]
  n292 = property on="Progress" class="Clust (strict)"("Visible"=w27) -> ()  [unwired: 2 in, 2 out]
  n293 = property on="Test Ring" class="Ring (strict)"("Visible"=w27) -> ()  [unwired: 2 in, 2 out]
  n294 = property on="Rev/Fwd" class="Clust (strict)"("Visible"=w27) -> ()  [unwired: 2 in, 2 out]
  n295 = property on="Camera Settings" class="Clust (strict)"("Visible"=w27) -> ()  [unwired: 2 in, 2 out]
  n296 = local write "DB Camera Config"(w27) -> ()
  n297 = global write "WPI_DashboardLogging Global.vi" "Recording"(w10) -> ()
  n298 = local write "Rec Mode"(w10) -> ()
